vi "Max_of_3.vi"(8 "error in (no error)":errorcluster, 9 "input 2":dbl, 10 "input 3":dbl, 11 "input 1":dbl) -> (0 "error out":errorcluster, 3 "Numeric out":dbl)   [LabVIEW 2022 SP3]
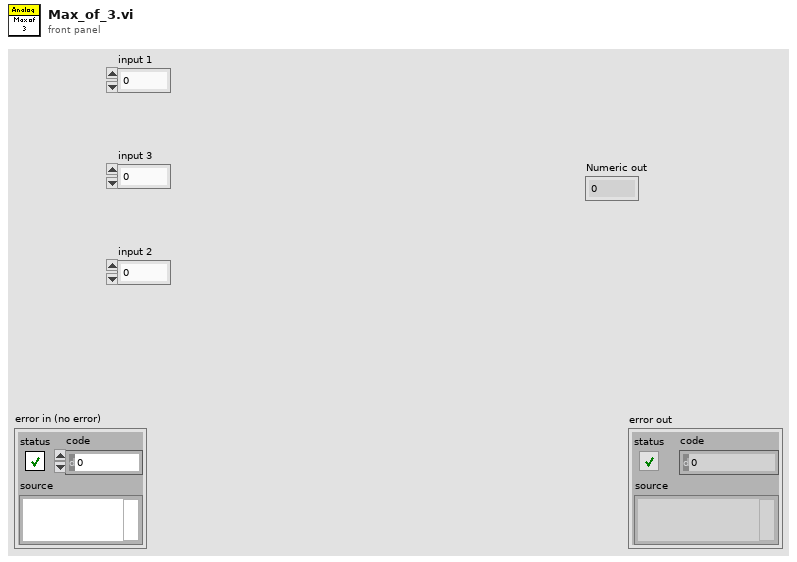
[diagram p1: front panel]
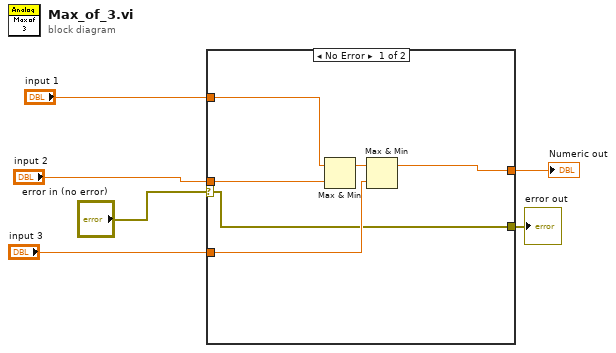
[diagram p0: block diagram]
diagram:
  n1 = case shown="No Error" "error in (no error)" {
    selector: "error in (no error)" -> [w7 w13]
    tunnel: "input 1" -> [w12 _]
    tunnel: "input 3" -> [w11 _]
    tunnel: [w10 _] -> w4
    tunnel: "input 2" -> [w9 _]
    tunnel: [w7 w13] -> w1
    frame No Error {
      n2 = Max & Min(x=w12, y=w9) -> (max(x,y)=w8:dbl)  [unwired: 1 out]
      n3 = Max & Min(x=w8, y=w11) -> (max(x,y)=w10:dbl)  [unwired: 1 out]
    }
    frame Error {
    }
  }
  "Numeric out" <- w4
  "error out" <- w1
